vi "UI Initialize.vi"(8 "error in (no error)":errorcluster, 11 "TestBench in":refnum<class "TestBench.lvclass">) -> (0 "error out":errorcluster, 3 "TestBench out":refnum<class "TestBench.lvclass">)   [LabVIEW 2019, in "TestBench.lvlib" / "TestBench.lvclass"]
uses:
  TestBench.lvclass
  TestBench.lvclass/TestBench.ctl
  <vilib>/ActorFramework/Message Enqueuer/Message Enqueuer.lvclass/Message Enqueuer.ctl
  <vilib>/ActorFramework/Message Enqueuer/Enqueue.vi
  SystemSetup/SystemSetup Messages/RefreshSystemConfigurationUI Msg/RefreshSystemConfigurationUI Msg.lvclass
  C:/Program Files (x86)/National Instruments/LabVIEW 2019/vi.lib/ActorFramework/Message/Message.lvclass
  SignalProcessing/SignalProcessing/SignalProcessing Global.vi
  <vilib>/ActorFramework/Message Priority Queue/Priority Enqueue.vi
  SignalProcessing/SignalProcessing/SignalProcessing.lvclass
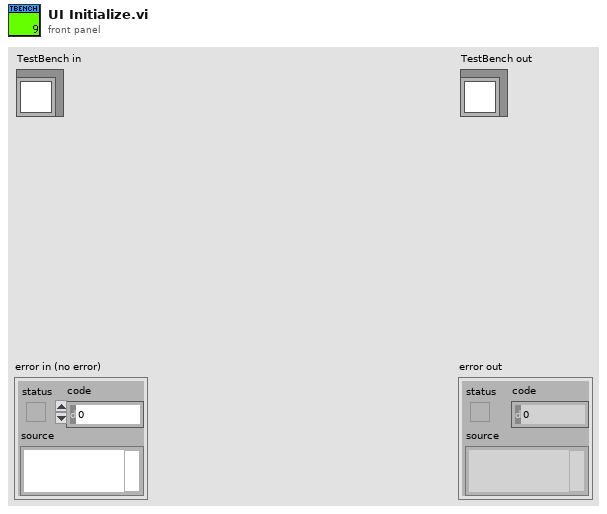
[diagram p1: front panel]
types:
  T1 = enum16{"Station 1", "Station 2", "Station 3", "Station 4"}[]
  T2 = enum16{"Station 1", "Station 2", "Station 3", "Station 4"}
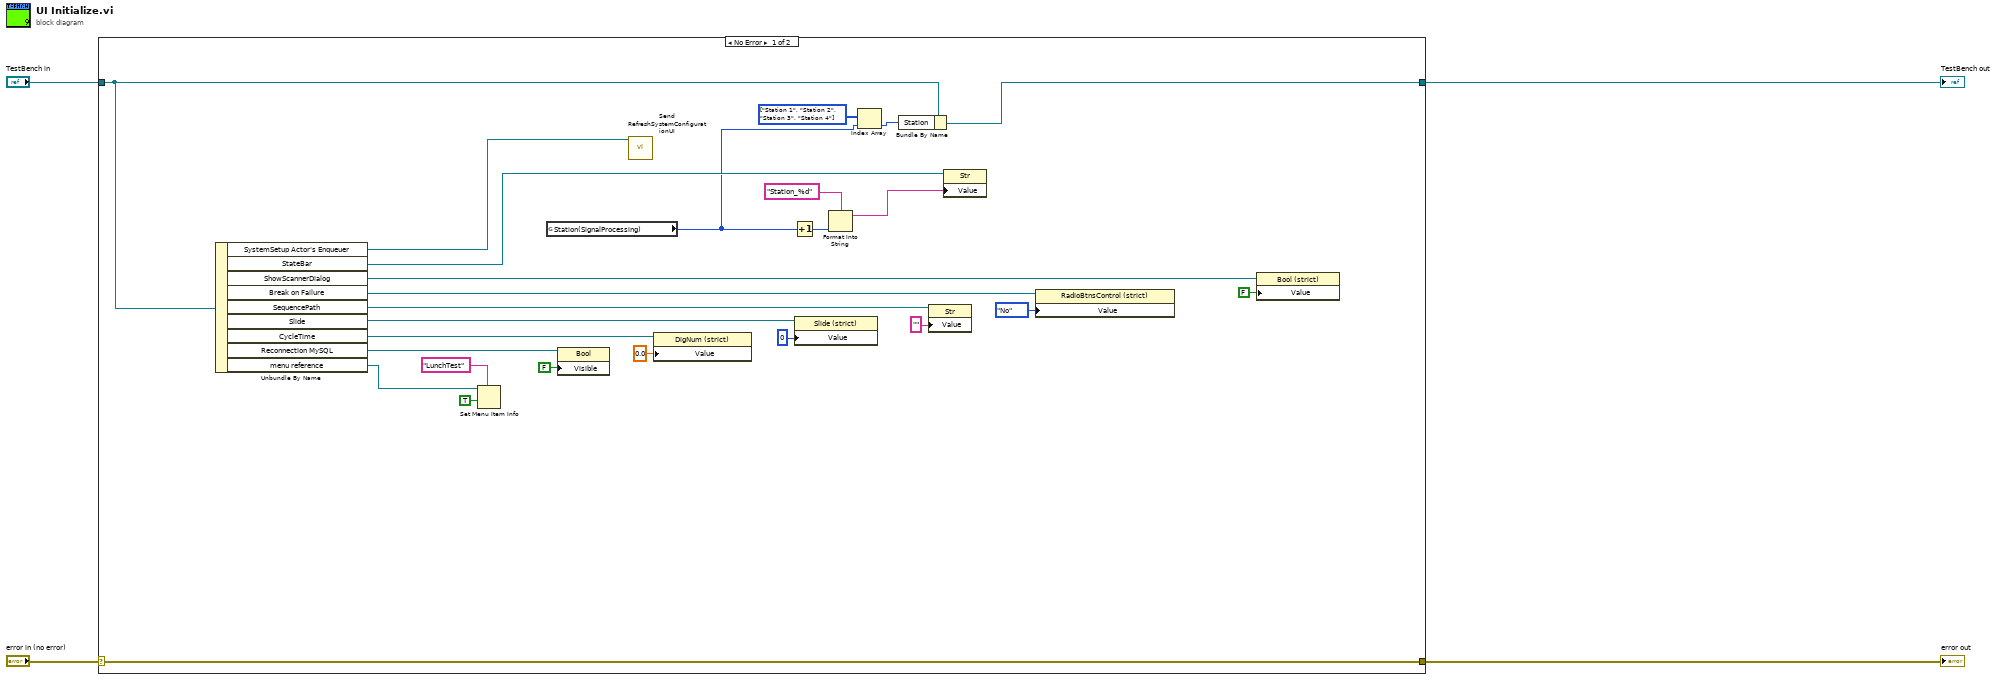
[diagram p0: block diagram]
diagram:
  n1 = case shown="No Error" "error in (no error)" {
    selector: "error in (no error)" -> [w30 w32]
    tunnel: [w30 w32] -> w3
    tunnel: [w6 w31] -> w1
    tunnel: "TestBench in" -> [w10 w31]
    frame No Error {
      w9 = T1 [enum."Station 1", enum."Station 2", enum."Station 3", enum."Station 4"] items=["Station 1", "Station 2", "Station 3", "Station 4"]
      n2 = Unbundle By Name(w10) -> ("SystemSetup Actor's Enqueuer"=w5:refnum<class "Message Enqueuer.lvclass">, "StateBar"=w14:refnum<vi>, "ShowScannerDialog"=w21:refnum<vi>, "Break on Failure"=w23:refnum<vi>, "SequencePath"=w25:refnum<vi>, "Slide"=w27:refnum<vi>, "CycleTime"=w29:refnum<vi>, "Reconnection MySQL"=w19:refnum<vi>, "menu reference"=w15:refnum<k9>)
      n3 = Set Menu Item Info(7:"LunchTest" ("item tag"), 9:TRUE ("enabled"), 11:w15) -> ()  [unwired: 4 in, 2 out]
      n4 = global read "SignalProcessing Global.vi" "Station(SignalProcessing)"() -> (w8:i32)
      n5 = property class="Bool"(reference=w19, "Visible"=FALSE) -> ()  [unwired: 1 in, 2 out]
      n6 = call "Send RefreshSystemConfigurationUI.vi"("Message Enqueuer"=w5) -> ()  [unwired: 9 in, 2 out]
      n7 = property class="DigNum (strict)"(reference=w29, "Value"=0.0) -> ()  [unwired: 1 in, 2 out]
      n8 = Increment(x=w8) -> (x+1=w11:i32)
      n9 = property class="Slide (strict)"(reference=w27, "Value"=u32 0) -> ()  [unwired: 1 in, 2 out]
      n10 = Format Into String(format string="Station_%d", w11) -> (resulting string=w12:string)  [unwired: 2 in, 1 out]
      n11 = Index Array(array=w9, index=w8) -> (element=w7:T2)
      n12 = Bundle By Name(cluster=w10, "Station"=w7) -> (w6:refnum<class "TestBench.lvclass">)
      n13 = property class="Str"(reference=w25, "Value"="") -> ()  [unwired: 1 in, 2 out]
      n14 = property class="Str"(reference=w14, "Value"=w12) -> ()  [unwired: 1 in, 2 out]
      n15 = property class="RadioBtnsControl (strict)"(reference=w23, "Value"=enum32{"Yes", "No"}."No") -> ()  [unwired: 1 in, 2 out]
      n16 = property class="Bool (strict)"(reference=w21, "Value"=FALSE) -> ()  [unwired: 1 in, 2 out]
    }
    frame Error {
    }
  }
  "error out" <- w3
  "TestBench out" <- w1
